vi "M Solar cells.vi"(11 "EV3 in":T1) -> (3 "EV3 out":T1)   [LabVIEW 2016]
uses:
  <vilib>/NXT/Subs/LVHSConnector.ctl
  <vilib>/NXT/LegoClasses/BrickReference/BrickReference.lvclass
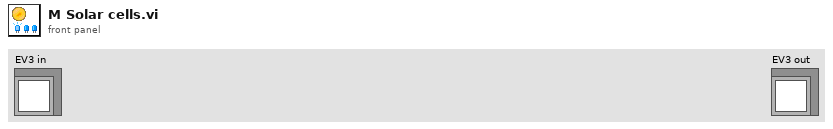
[diagram p1: front panel]
types:
  T1 = typedef "LVHSConnector.ctl" = refnum<class "BrickReference.lvclass">
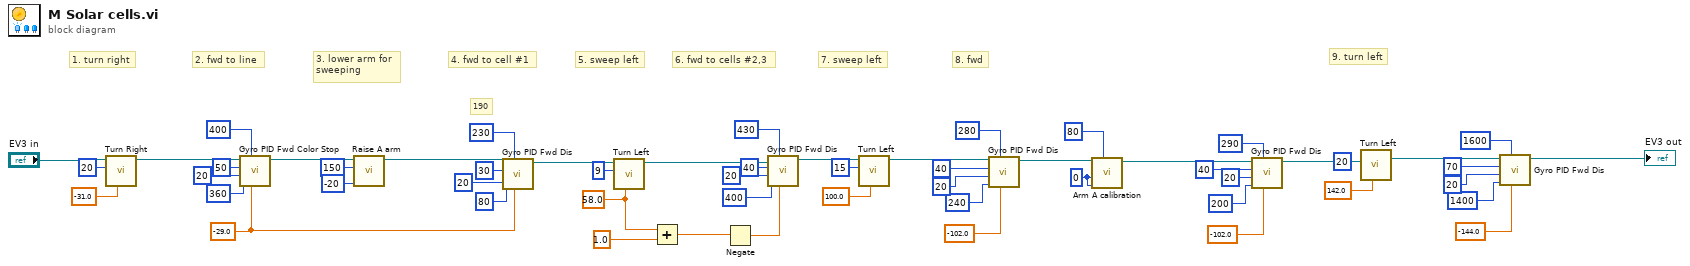
[diagram p0: block diagram]
diagram:
  w11 = 0 ("Rotation")
  w35 = sgl 58.0 ("Turning angle")
  w41 = sgl -29.0 ("Target angle")
  # "190"
  # "9. turn left"
  # "8. fwd"
  # "7. sweep left"
  # "6. fwd to cells #2,3"
  # "5. sweep left"
  # "4. fwd to cell #1"
  # "3. lower arm for\nsweeping"
  # "2. fwd to line"
  # "1. turn right"
  n1 = call "Turn Right.vi"("Turning angle"=sgl -31.0, "Motor B (right)"=i8 20, "EV3 in"="EV3 in") -> ("EV3 out"=w55:T1)  [unwired: 8 in]
  n2 = call "Gyro PID Fwd Color Stop.vi"("Target angle"=w41, "Threshold to Color"=400 ("Threshold to stop"), "Threshold to slow"=360, "Min. speed"=20, "Max. speed"=50, "EV3 in"=w55) -> ("EV3 out"=w48:T1)  [unwired: 5 in]
  n3 = call "Raise A arm.vi"("Power"=i8 -20, "Rotation"=150, "EV3 in"=w48) -> ("EV3 out"=w42:T1)  [unwired: 8 in]
  n4 = call "Gyro PID Fwd Dis.vi"("Target angle"=w41, "Threshold to stop"=230, "Threshold to slow"=80, "Min. speed"=20, "Max. speed"=30, "EV3 in"=w42) -> ("EV3 out"=w40:T1)  [unwired: 5 in]
  n5 = call "Turn Left.vi"("Turning angle"=w35, "Motor B (right)"=i8 9, "EV3 in"=w40) -> ("EV3 out"=w38:T1)  [unwired: 8 in]
  n6 = Add(x=w35, y=sgl 1.0) -> (x+y=w34:sgl)
  n7 = Negate(x=w34) -> (-x=w32:sgl)
  n8 = call "Gyro PID Fwd Dis.vi"("Target angle"=w32, "Threshold to stop"=430, "Threshold to slow"=400, "Min. speed"=20, "Max. speed"=40, "EV3 in"=w38) -> ("EV3 out"=w28:T1)  [unwired: 5 in]
  n9 = call "Turn Left.vi"("Turning angle"=sgl 100.0, "Motor B (right)"=i8 15, "EV3 in"=w28) -> ("EV3 out"=w22:T1)  [unwired: 8 in]
  n10 = call "Gyro PID Fwd Dis.vi"("Target angle"=sgl -102.0, "Threshold to stop"=280, "Threshold to slow"=240, "Min. speed"=20, "Max. speed"=40, "EV3 in"=w22) -> ("EV3 out"=w19:T1)  [unwired: 5 in]
  n11 = call "Arm A calibration.vi"("Cali. Power"=i8 80, "Down Power"=w11, "Rotation"=w11, "NXT/EV3"=w19) -> ("NXT/EV3"=w13:T1)  [unwired: 7 in]
  n12 = call "Gyro PID Fwd Dis.vi"("Target angle"=sgl -102.0, "Threshold to stop"=290, "Threshold to slow"=200, "Min. speed"=20, "Max. speed"=40, "EV3 in"=w13) -> ("EV3 out"=w10:T1)  [unwired: 5 in]
  n13 = call "Turn Left.vi"("Turning angle"=sgl 142.0, "Motor B (right)"=i8 20, "EV3 in"=w10) -> ("EV3 out"=w2:T1)  [unwired: 8 in]
  n14 = call "Gyro PID Fwd Dis.vi"("Target angle"=sgl -144.0, "Threshold to stop"=1600, "Threshold to slow"=1400, "Min. speed"=20, "Max. speed"=70, "EV3 in"=w2) -> ("EV3 out"=→"EV3 out":T1)  [unwired: 5 in]
